vi "Get Cell String.vi"(8 "error in":errorcluster, 9 "Cell Address":string, 10 "Sheet Name":string, 11 "OpenXml in":refnum<class "OpenXml.lvclass">) -> (0 "error out":errorcluster, 2 "Value String":string, 3 "OpenXml out":refnum<class "OpenXml.lvclass">)   [LabVIEW 2024, in "OpenXml.lvclass"]
uses:
  OpenXml.lvclass
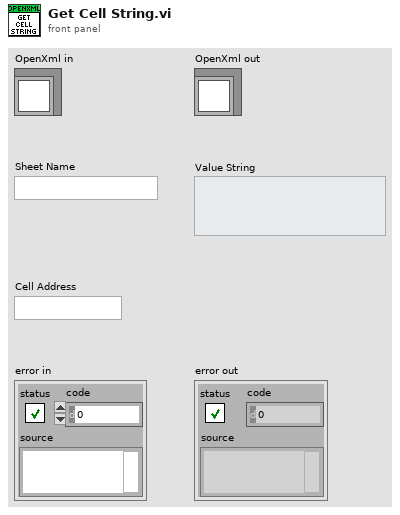
[diagram p1: front panel]
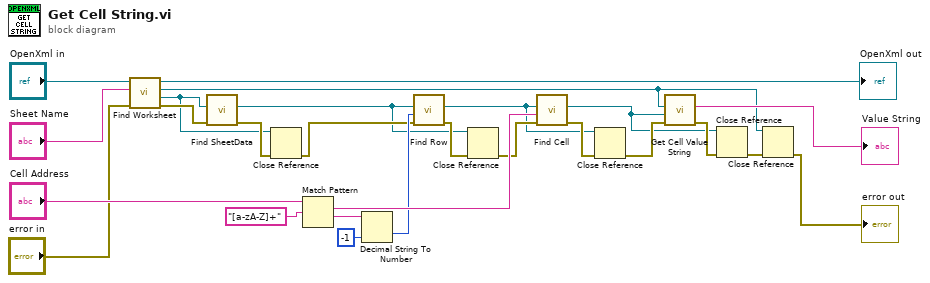
[diagram p0: block diagram]
diagram:
  n1 = call "Find Worksheet.vi"("error in"="error in", "Sheet Name"="Sheet Name", "OpenXml in"="OpenXml in") -> ("error out"=w23:errorcluster, "Worksheet"=w9:refnum<k24>, "WorkbookPart"=w1:refnum<k24>, "OpenXml out"=→"OpenXml out":refnum<class "OpenXml.lvclass">)  [unwired: 5 in]
  n2 = call "Find SheetData.vi"("error in"=w23, "Worksheet"=w9) -> ("error out"=w14:errorcluster, "SheetData"=w7:refnum<k24>)  [unwired: 8 in]
  n3 = Close Reference(reference=w9, error in (no error)=w14) -> (error out=w10:errorcluster)
  n4 = Match Pattern(string="Cell Address", regular expression="[a-zA-Z]+") -> (match substring=w20:string, after substring=w19:string)  [unwired: 1 in, 2 out]
  n5 = Decimal String To Number(string=w19, default (0L)=-1 ("default (0 I32)")) -> (number=w18:i32)  [unwired: 1 in, 1 out]
  n6 = call "Find Row.vi"("error in"=w10, "Index"=w18, "SheetData"=w7) -> ("error out"=w12:errorcluster, "Row"=w5:refnum<k24>)  [unwired: 7 in]
  n7 = Close Reference(reference=w7, error in (no error)=w12) -> (error out=w8:errorcluster)
  n8 = call "Find Cell.vi"("error in"=w8, "Lexical Index"=w20, "Row"=w5) -> ("error out"=w13:errorcluster, "Cell"=w2:refnum<k24>)  [unwired: 7 in]
  n9 = Close Reference(reference=w5, error in (no error)=w13) -> (error out=w6:errorcluster)
  n10 = call "Get Cell Value String.vi"("error in"=w6, "Cell"=w2, "Workbookpart"=w1) -> ("error out"=w16:errorcluster, "Value String"=→"Value String":string)  [unwired: 7 in]
  n11 = Close Reference(reference=w2, error in (no error)=w16) -> (error out=w4:errorcluster)
  n12 = Close Reference(reference=w1, error in (no error)=w4) -> (error out=→"error out":errorcluster)
